vi "MEMS Path.vi"() -> (2 "stripped path":path)   [LabVIEW 2014]
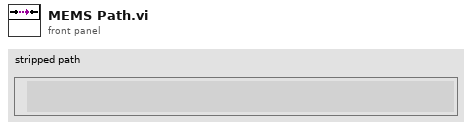
[diagram p1: front panel]
types:
  T1 = enum32{"invalid app kind", "Development System", "Run Time System", "Student Edition", "Embedded LabVIEW", "Evaluation", "Custom"}
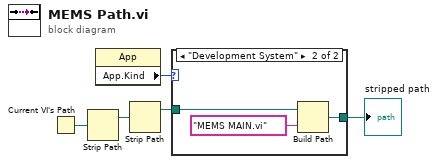
[diagram p0: block diagram]
diagram:
  n1 = Current VI's Path() -> (path=w5:path)
  n2 = Strip Path(path=w5) -> (stripped path=w2:path)  [unwired: 1 out]
  n3 = property class="App"() -> ("App.Kind"=w4:T1)  [unwired: 2 in, 2 out]
  n4 = Strip Path(path=w2) -> (stripped path=w3:path)  [unwired: 1 out]
  n5 = case shown="\"Development System\"" w4 {
    tunnel: w3 -> [_ w8]
    tunnel: [_ w6] -> w1
    frame "invalid app kind", Default {
    }
    frame "Development System" {
      n6 = Build Path(base path=w8, name or relative path="MEMS MAIN.vi" ("名称或相对路径")) -> (appended path=w6:path)
    }
  }
  "stripped path" <- w1
